vi "PV 2 Data.vi"(3 "Error In":errorcluster, 5 "PV":refnum<class "PV.lvclass">) -> (0 "Error Out":errorcluster, 1 "Data":string, 2 "Quality":i32)   [LabVIEW 2014, in "CS++DIM.lvlib" / "DIMConnection.lvclass"]
doc: "Convert PV variant data to byte array (string)."
uses:
  DIMConnection.lvclass
  CSPP_Core/Classes/CS++ProcessVariables/ProcessVariable/PV.lvclass
  CSPP_Core/Libraries/Utilities/CS++Utilities.lvlib
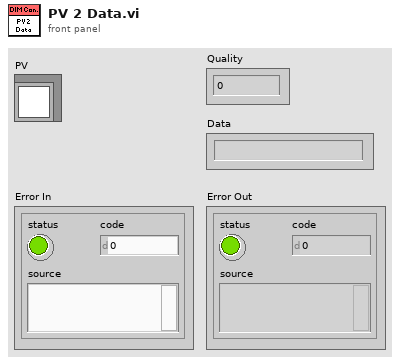
[diagram p1: front panel]
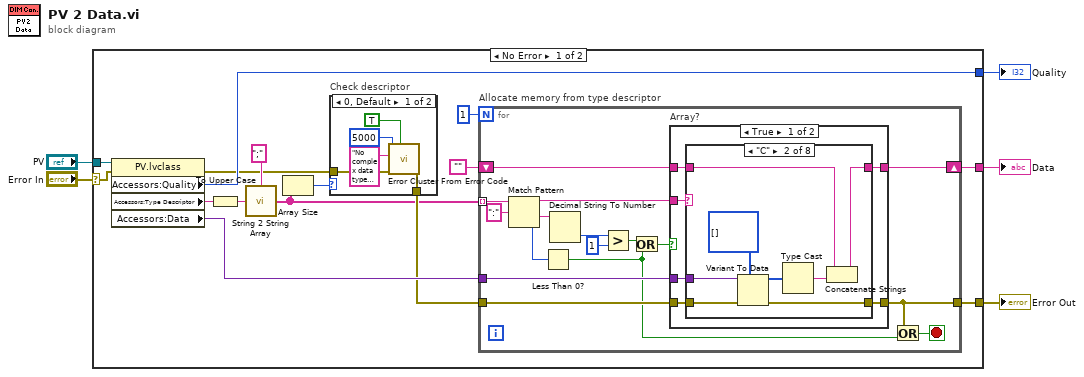
[diagram p0: block diagram]
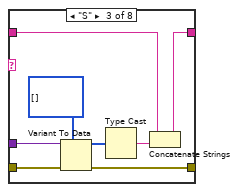
[diagram p4: hidden frame]
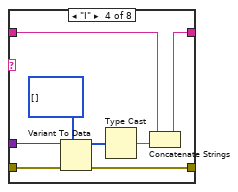
[diagram p5: hidden frame]
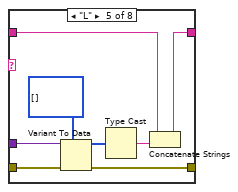
[diagram p6: hidden frame]
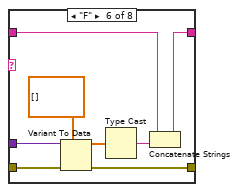
[diagram p7: hidden frame]
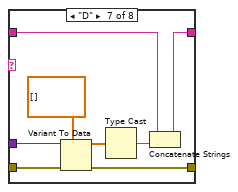
[diagram p8: hidden frame]
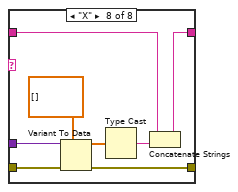
[diagram p9: hidden frame]
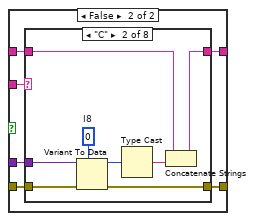
[diagram p10: hidden frame]
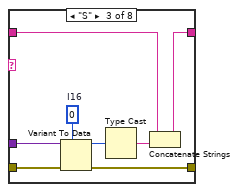
[diagram p12: hidden frame]
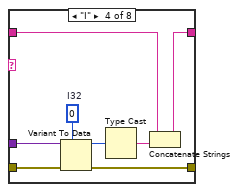
[diagram p13: hidden frame]
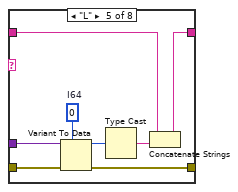
[diagram p14: hidden frame]
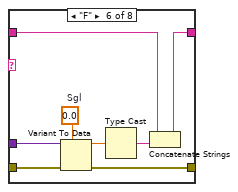
[diagram p15: hidden frame]
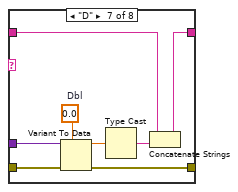
[diagram p16: hidden frame]
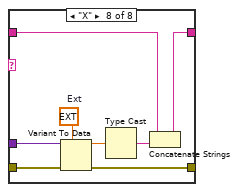
[diagram p17: hidden frame]
diagram:
  n1 = case shown="No Error" "Error In" {
    selector: "Error In" -> [w6 w171]
    tunnel: [w18 _] -> w5
    tunnel: "PV" -> [w16 _]
    tunnel: [w14 _] -> w3
    tunnel: [w12 w171] -> w2
    frame No Error {
      n2 = property class="PV.lvclass"(reference=w16, error in=w6) -> (error out=w10:errorcluster, "Accessors:Quality"=w14:i32, "Accessors:Type Descriptor"=w15:string, "Accessors:Data"=w13:variant)  [unwired: 1 out]
      n3 = To Upper Case(1:w15) -> (0:w17:string)
      n4 = call "String 2 String Array.vi"("String"=w17, "Delimiter (\",\")"=";" ("Delimiter (\",\")")) -> ("Substrings"=w8:string[])
      n5 = Array Size(array=w8) -> (size(s)=w7:i32)
      n6 = case "Check descriptor" shown="0, Default" w7 {
        tunnel: w10 -> [w25 w26]
        tunnel: [w24 w26] -> w9
        frame 0, Default {
          n7 = call <vilib>:"Error Cluster From Error Code.vi"("show call chain? (False)"=TRUE, "error in (no error)"=w25, "error message (\"\")"="No complex data types support for now." ("error message (\"\")"), "error code (0)"=5000) -> ("error out"=w24:errorcluster)  [unwired: 5 in]
        }
        frame 1 {
        }
      }
      n8 = for "Allocate memory from type descriptor" {
        N: 1 -> [_]
        tunnel: w8 -> [w42] mode=indexing
        shift-right: [w38] -> w18
        shift-left: "" -> [w40]
        tunnel: w13 -> [w37]
        tunnel: w9 -> [w30]
        tunnel: [w28] -> w12
        stop <- w29 stop-if-true
        n9 = Match Pattern(string=w42, regular expression=":") -> (before substring=w39:string, after substring=w35:string, offset past match=w36:i32)  [unwired: 1 in, 1 out]
        n10 = Less Than 0?(x=w36) -> (x < 0?=w27:bool)
        n11 = Decimal String To Number(string=w35) -> (number=w34:i32)  [unwired: 2 in, 1 out]
        n12 = Greater?(x=w34, y=1) -> (0:w32:bool)
        n13 = Or(x=w32, y=w27) -> (x .or. y?=w31:bool)
        n14 = case "Array?" shown="True" w31 {
          tunnel: w40 -> [w48 w112]
          tunnel: w39 -> [w47 w111]
          tunnel: [w46 w110] -> w38
          tunnel: w37 -> [w45 w109]
          tunnel: w30 -> [w44 w108]
          tunnel: [w43 w107] -> w28
          frame True {
            n15 = case shown="\"C\"" w47 {
              tunnel: w48 -> [w50 w54 w62 w70 w78 w86 w94 w102]
              tunnel: [w50 w53 w61 w69 w77 w85 w93 w101] -> w46
              tunnel: w45 -> [_ w58 w66 w74 w82 w90 w98 w106]
              tunnel: w44 -> [w49 w57 w65 w73 w81 w89 w97 w105]
              tunnel: [w49 w51 w59 w67 w75 w83 w91 w99] -> w43
              frame Default {
              }
              frame "C" {
                n16 = Variant To Data(error in=w57, type=i8[] [], Variant=w58) -> (data=w52:i8[], error out=w51:errorcluster)
                n17 = Type Cast(x=w52) -> (*(type *) &x=w55:string)  [unwired: 1 in]
                n18 = Concatenate Strings(w54, w55) -> (w53:string)
              }
              frame "S" {
                n19 = Variant To Data(error in=w65, type=i16[] [], Variant=w66) -> (data=w60:i16[], error out=w59:errorcluster)
                n20 = Type Cast(x=w60) -> (*(type *) &x=w63:string)  [unwired: 1 in]
                n21 = Concatenate Strings(w62, w63) -> (w61:string)
              }
              frame "I" {
                n22 = Variant To Data(error in=w73, type=i32[] [], Variant=w74) -> (data=w68:i32[], error out=w67:errorcluster)
                n23 = Type Cast(x=w68) -> (*(type *) &x=w71:string)  [unwired: 1 in]
                n24 = Concatenate Strings(w70, w71) -> (w69:string)
              }
              frame "L" {
                n25 = Variant To Data(error in=w81, type=i64[] [], Variant=w82) -> (data=w76:i64[], error out=w75:errorcluster)
                n26 = Type Cast(x=w76) -> (*(type *) &x=w79:string)  [unwired: 1 in]
                n27 = Concatenate Strings(w78, w79) -> (w77:string)
              }
              frame "F" {
                n28 = Variant To Data(error in=w89, type=sgl[] [], Variant=w90) -> (data=w84:sgl[], error out=w83:errorcluster)
                n29 = Type Cast(x=w84) -> (*(type *) &x=w87:string)  [unwired: 1 in]
                n30 = Concatenate Strings(w86, w87) -> (w85:string)
              }
              frame "D" {
                n31 = Variant To Data(error in=w97, type=dbl[] [], Variant=w98) -> (data=w92:dbl[], error out=w91:errorcluster)
                n32 = Type Cast(x=w92) -> (*(type *) &x=w95:string)  [unwired: 1 in]
                n33 = Concatenate Strings(w94, w95) -> (w93:string)
              }
              frame "X" {
                n34 = Variant To Data(error in=w105, type=ext[] [], Variant=w106) -> (data=w100:ext[], error out=w99:errorcluster)
                n35 = Type Cast(x=w100) -> (*(type *) &x=w103:string)  [unwired: 1 in]
                n36 = Concatenate Strings(w102, w103) -> (w101:string)
              }
            }
          }
          frame False {
            n37 = case shown="\"C\"" w111 {
              tunnel: w112 -> [w114 w119 w127 w135 w143 w151 w159 w167]
              tunnel: [w114 w118 w126 w134 w142 w150 w158 w166] -> w110
              tunnel: w109 -> [_ w122 w130 w138 w146 w154 w162 w170]
              tunnel: w108 -> [w113 w121 w129 w137 w145 w153 w161 w169]
              tunnel: [w113 w116 w124 w132 w140 w148 w156 w164] -> w107
              frame Default {
              }
              frame "C" {
                w115 = i8 0  # I8
                n38 = Variant To Data(error in=w121, type=w115, Variant=w122) -> (data=w117:i8, error out=w116:errorcluster)
                n39 = Type Cast(x=w117) -> (*(type *) &x=w120:string)  [unwired: 1 in]
                n40 = Concatenate Strings(w119, w120) -> (w118:string)
              }
              frame "S" {
                w123 = i16 0  # I16
                n41 = Variant To Data(error in=w129, type=w123, Variant=w130) -> (data=w125:i16, error out=w124:errorcluster)
                n42 = Type Cast(x=w125) -> (*(type *) &x=w128:string)  [unwired: 1 in]
                n43 = Concatenate Strings(w127, w128) -> (w126:string)
              }
              frame "I" {
                w131 = 0  # I32
                n44 = Variant To Data(error in=w137, type=w131, Variant=w138) -> (data=w133:i32, error out=w132:errorcluster)
                n45 = Type Cast(x=w133) -> (*(type *) &x=w136:string)  [unwired: 1 in]
                n46 = Concatenate Strings(w135, w136) -> (w134:string)
              }
              frame "L" {
                w139 = i64 0  # I64
                n47 = Variant To Data(error in=w145, type=w139, Variant=w146) -> (data=w141:i64, error out=w140:errorcluster)
                n48 = Type Cast(x=w141) -> (*(type *) &x=w144:string)  [unwired: 1 in]
                n49 = Concatenate Strings(w143, w144) -> (w142:string)
              }
              frame "F" {
                w147 = sgl 0.0  # Sgl
                n50 = Variant To Data(error in=w153, type=w147, Variant=w154) -> (data=w149:sgl, error out=w148:errorcluster)
                n51 = Type Cast(x=w149) -> (*(type *) &x=w152:string)  [unwired: 1 in]
                n52 = Concatenate Strings(w151, w152) -> (w150:string)
              }
              frame "D" {
                w155 = 0.0  # Dbl
                n53 = Variant To Data(error in=w161, type=w155, Variant=w162) -> (data=w157:dbl, error out=w156:errorcluster)
                n54 = Type Cast(x=w157) -> (*(type *) &x=w160:string)  [unwired: 1 in]
                n55 = Concatenate Strings(w159, w160) -> (w158:string)
              }
              frame "X" {
                w163 = ext 0.0  # Ext
                n56 = Variant To Data(error in=w169, type=w163, Variant=w170) -> (data=w165:ext, error out=w164:errorcluster)
                n57 = Type Cast(x=w165) -> (*(type *) &x=w168:string)  [unwired: 1 in]
                n58 = Concatenate Strings(w167, w168) -> (w166:string)
              }
            }
          }
        }
        n59 = Or(x=w28, y=w27) -> (x .or. y?=w29:bool)
      }
    }
    frame Error {
    }
  }
  "Data" <- w5
  "Quality" <- w3
  "Error Out" <- w2
